vi "Host Main.vi"() -> ()   [LabVIEW 2013]
uses:
  <vilib>/NI/Module Execution Interface/Engine Runtime/Engine Runtime Interface.lvclass
  <vilib>/NI/Module Execution Interface/Engine Runtime/Execution States.ctl
  <vilib>/NI/Tag Bus Data Framework/Framework Configuration Classes/target runtime/PL_Target Runtime.lvclass
  <vilib>/NI/Configuration Framework/tree serializer/NISE_CEF_TreeSerializer.lvlib
  <vilib>/NI/Tag Bus Data Framework/Framework Configuration Classes/flattened data interface/PL_Serialization Interface.lvlib
panel:
  in  "target":i32
  in  "config. file path":path=path "C:/TBDF/Sample Applications/RT Temperature Controller/Host Simulation Configuration.pcfg"
  out "final error":errorcluster
  in  "stop":bool
  out "engine error":errorcluster
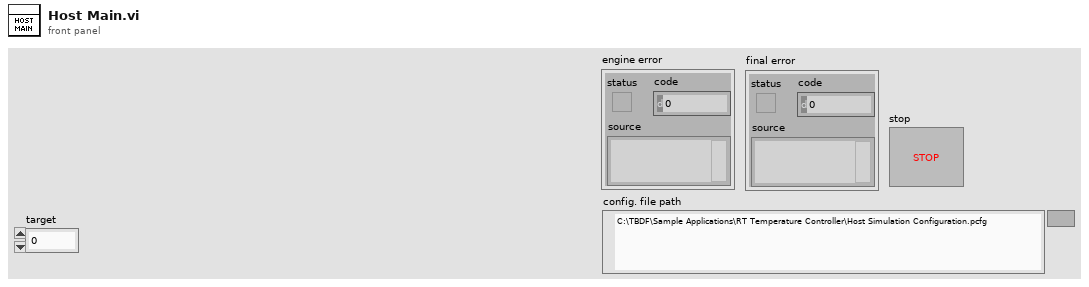
[diagram p1: front panel]
types:
  T1 = typedef "NISE_CEF_TreeSerializer.lvlib/base file format.ctl" = cluster{"version":string, "data":string}
  T2 = typedef "NISE_CEF_TreeSerializer.lvlib/flat hierarchy.ctl" = cluster{"hierarchy structure":T3, "instance data":T5[]}
  T3 = typedef "NISE_CEF_TreeSerializer.lvlib/full hierarchy.ctl" = cluster{"root":string, "hierarchy":T4[]}
  T4 = typedef "NISE_CEF_TreeSerializer.lvlib/hierarchy element.ctl" = cluster{"current node":string, "children":string[]}
  T5 = typedef "NISE_CEF_TreeSerializer.lvlib/instance data.ctl" = cluster{"ID":string, "Alias":string, "class":string, "version":string, "data":string}
  T6 = typedef "PLConfigurationSerializer.lvlib/targets cluster.ctl" = cluster{"Target Configuration":refnum<class "PL_Target Configuration.lvclass">, "engines":T7[]}
  T7 = typedef "PLConfigurationSerializer.lvlib/engines cluster.ctl" = cluster{"engine configuration":refnum<class "engine configuration.lvclass">, "modules":refnum<class "TBM module configuration.lvclass">[]}
  T8 = typedef "Engine Runtime Interface.lvclass/Execution States.ctl" = enum16{"Initializing", "Paused (Initialized)", "Running", "Set Safe Outputs", "Uninitializing", "Stopped (Uninitialized)", "Error (Uninitialized)", "Safe State (Uninitialized)", "Closed"}
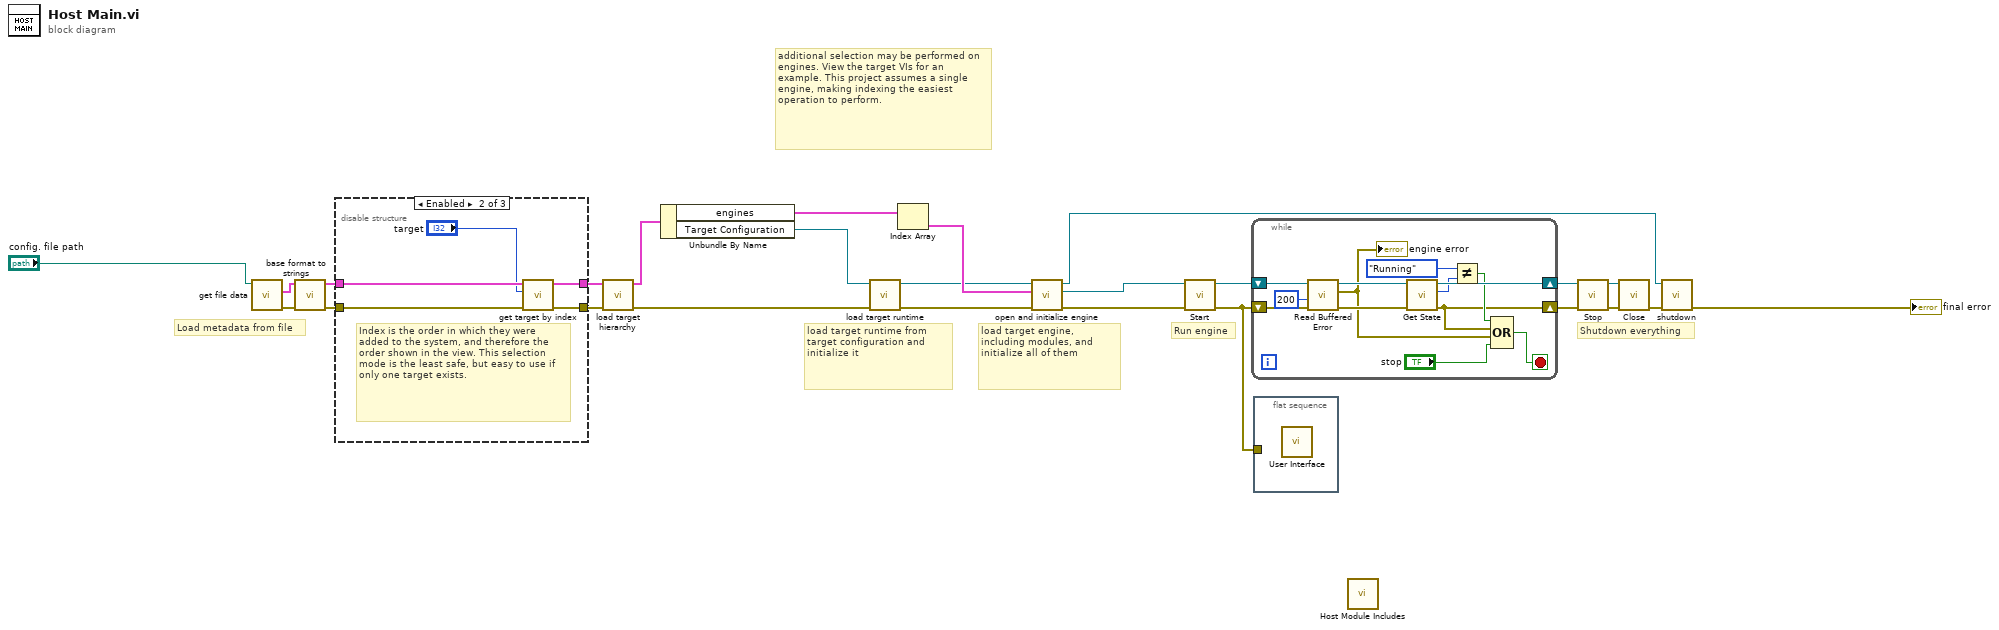
[diagram p0: block diagram]
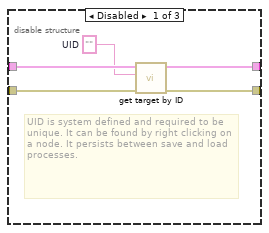
[diagram p2: hidden frame]
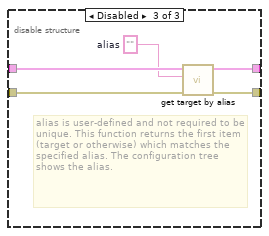
[diagram p3: hidden frame]
diagram:
  # "additional selection may be performed on engines. View the target VIs for an example. This project assumes a single engine, making indexing the easiest operation to perform."
  # "load target engine, including modules, and initialize all of them"
  # "load target runtime from target configuration and initialize it"
  # "Load metadata from file"
  # "Shutdown everything"
  # "Run engine"
  n1 = call <vilib>:"get file data.vi"("Path"="config. file path") -> ("error out"=w12:errorcluster, "format"=w11:T1)  [unwired: 9 in]
  n2 = call <vilib>:"base format to strings.vi"("error in"=w12, "format"=w11) -> ("error out"=w10:errorcluster, "data"=w9:T2)  [unwired: 8 in]
  n3 = disable-structure shown="Enabled" {
    disable-tunnel: w10 -> [w29 w32 w37]
    disable-tunnel: w9 -> [w30 w33 w38]
    disable-tunnel: [w27 w35 w40] -> w8
    disable-tunnel: [w26 w34 w39] -> w7
    frame Disabled {
      w28 = ""  # UID
      # "UID is system defined and required to be unique. It can be found by right clicking on a node. It persists between save and load processes."
      n4 = call <vilib>:"get target by ID.vi"("error in"=w29, "UID"=w28, "full system"=w30) -> ("error out"=w26:errorcluster, "target hierarchy"=w27:T2)  [unwired: 7 in]
    }
    frame Enabled {
      # "Index is the order in which they were added to the system, and therefore the order shown in the view. This selection mode is the least safe, but easy to use if only one target exists."
      n5 = call <vilib>:"get target by index.vi"("error in"=w32, "index"="target", "system hierarchy"=w33) -> ("error out"=w34:errorcluster, "target hierarchy"=w35:T2)  [unwired: 7 in]
    }
    frame Disabled {
      w36 = ""  # alias
      # "alias is user-defined and not required to be unique. This function returns the first item (target or otherwise) which matches the specified alias. The configuration tree shows the alias."
      n6 = call <vilib>:"get target by alias.vi"("error in"=w37, "alias"=w36, "system hierarchy"=w38) -> ("error out"=w39:errorcluster, "target hierarchy"=w40:T2)  [unwired: 7 in]
    }
  }
  n7 = call <vilib>:"load target hierarchy.vi"("error in"=w7, "target hierarchy"=w8) -> ("error out"=w6:errorcluster, "targets cluster out"=w5:T6)  [unwired: 8 in]
  n8 = Unbundle By Name(w5) -> ("engines"=w17:T7[], "Target Configuration"=w15:refnum<class "PL_Target Configuration.lvclass">)
  n9 = call <vilib>:"load target runtime.vi"("error in"=w6, "target configuration"=w15) -> ("error out"=w14:errorcluster, "target runtime"=w13:refnum<class "PL_Target Runtime.lvclass">)  [unwired: 8 in]
  n10 = Index Array(array=w17) -> (element=w16:T7)  [unwired: 1 in]
  n11 = call <vilib>:"open and initialize engine.vi"("error in"=w14, "engine configuration in"=w16, "Target Runtime in"=w13) -> ("error out"=w3:errorcluster, "Engine Runtime Interface out"=w1:refnum<class "Engine Runtime Interface.lvclass">, "Target Runtime out"=w2:refnum<class "PL_Target Runtime.lvclass">)  [unwired: 6 in]
  n12 = call-dynamic "Start.vi"("error in"=w3, "Engine Runtime Interface in"=w1) -> ("error out"=w18:errorcluster, "Engine Runtime Interface out"=w23:refnum<class "Engine Runtime Interface.lvclass">)  [unwired: 8 in]
  n13 = while {
    shift-right: [w49] -> w22
    shift-left: w23 -> [w53]
    shift-right: [w42] -> w21
    shift-left: w18 -> [w52]
    stop <- w47 stop-if-true
    n14 = call-dynamic "Read Buffered Error.vi"("error in"=w52, "timeout in ms (0)"=200, "Engine Runtime Interface in"=w53) -> ("error out"=w50:errorcluster, "Engine Error"=w46:errorcluster, "Engine Runtime Interface out"=w51:refnum<class "Engine Runtime Interface.lvclass">)  [unwired: 6 in]
    "engine error" <- w46
    n15 = call-dynamic "Get State.vi"("error in"=w50, "Engine Runtime Interface in"=w51) -> ("error out"=w42:errorcluster, "Engine State"=w45:T8, "Engine Runtime Interface out"=w49:refnum<class "Engine Runtime Interface.lvclass">)  [unwired: 7 in]
    n16 = Not Equal?(x=Execution_States."Running" ("Engine State"), y=w45) -> (x != y?=w43:bool)
    n17 = Compound Arithmetic op=OR(w43, w42, w46, "stop") -> (w47:bool)
  }
  n18 = flat-sequence {
    tunnel: w18 -> [_]
    frame #0 {
      n19 = call "User Interface.vi"() -> ()  [unwired: 12 in]
    }
  }
  n20 = call "Host Module Includes.vi"() -> ()  [unwired: 12 in]
  n21 = call-dynamic "Stop.vi"("error in"=w21, "Engine Runtime Interface in"=w22) -> ("error out"=w24:errorcluster, "Engine Runtime Interface out"=w25:refnum<class "Engine Runtime Interface.lvclass">)  [unwired: 8 in]
  n22 = call-dynamic "Close.vi"("error in"=w24, "Engine Runtime Interface in"=w25) -> ("error out"=w20:errorcluster)  [unwired: 9 in]
  n23 = call-dynamic "shutdown.vi"("error in"=w20, "Target Runtime in"=w2) -> ("error out"=→"final error":errorcluster)  [unwired: 9 in]
